vi "Magnetic Sweep 1.9c.vi"() -> ()   [LabVIEW 2011]
panel:
  in  "Save":bool
  out "file position4":errorcluster
  out "file position3":errorcluster
  out "file position2":errorcluster
  out "File position1":errorcluster
  out "Initial Temperature check":errorcluster
  out "Status":i32
  out "Loop end check":errorcluster
  out "Parameter setup":errorcluster
  out "Resistance check":errorcluster
  out "Start ramping":errorcluster
  out "Cell temperature\ncheck":errorcluster
  out "Initial Temp\nCheck":errorcluster
  out "Current time":timestamp format="%<%I:%M:%S %p\n%x>T"
  out "x .and. y?":bool
  in  "Initial\nTemperature":dbl
  out "Heater":bool
  out "Persistent switch ready":bool
  out "Initial check":errorcluster
  in  "Temperature\nlower limite":dbl
  out "Ramping rate command":string
  out "Target field command":string
  out "String":string="Persistent switch is not on"
  in  "Set parameter":bool
  out "status":string
  out "PID command":string
  out "setpoint command":string
  out "setpoint":dbl
  in  "stop":bool
  in  "Contour plot (ramp down)":path
  in  "Raw data (ramp down)":path
  out "Elapsed Time (s)":dbl
  out "Iteration":i32
  out "Zero field reached":bool
  out "Target field reached":bool
  in  "Temperature\nupper limite":dbl
  in  "Temperature\nramping step":dbl
  in  "Heater range":i16(ring) items=["High", "Medium", "Low"]
  in  "D gain":dbl
  in  "I gain":dbl
  in  "P gain":dbl
  in  "Contour plot (ramp up)":path
  in  "Timer":bool caption="Reset"
  in  "Raw data (ramp  up)":path
  out "Current Resistance":string
  out "Current Temperature":string
  out "Current Field":string
  in  "Sweep":bool
  in  "Magnetic field\nRamp rate":dbl
  in  "Traget Field":dbl
  out "Init Response":string
  in  "Update":bool
  in  "P Switch on/off":bool
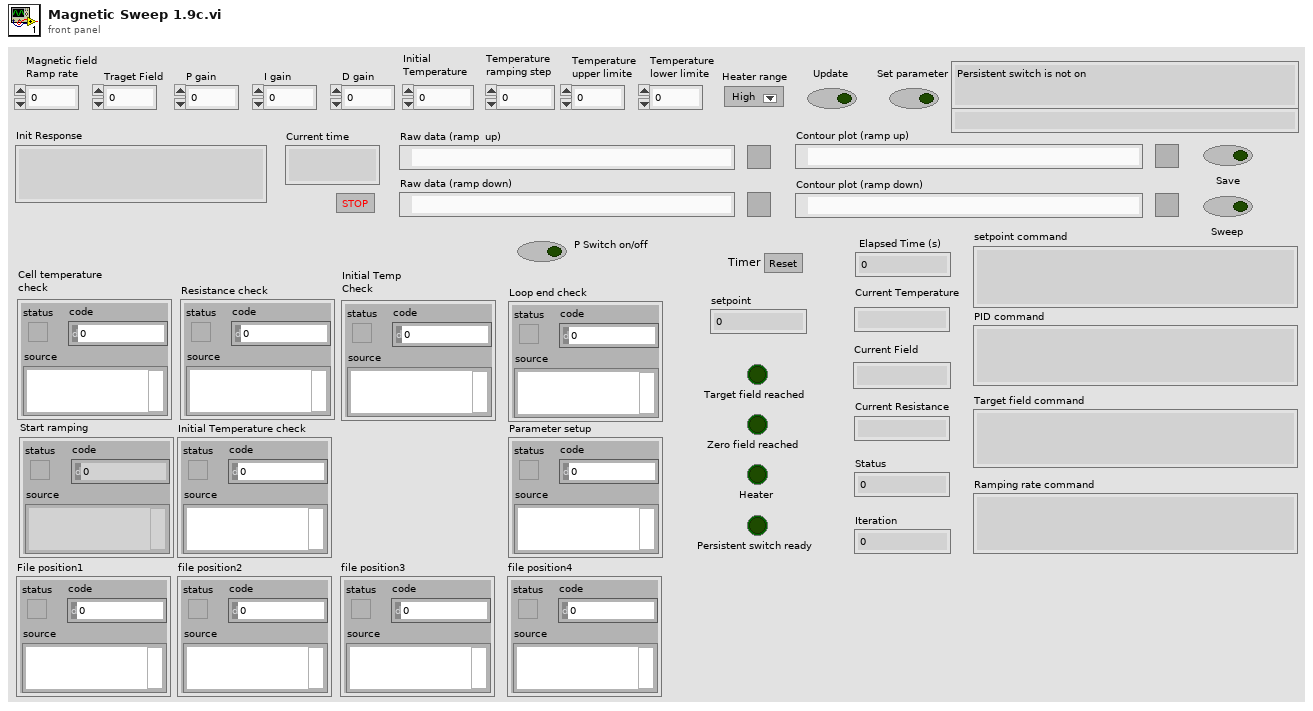
[diagram p1: front panel]
types:
  T1 = enum16{"open", "replace", "create", "open or create", "replace or create", "replace or create with confirmation"}
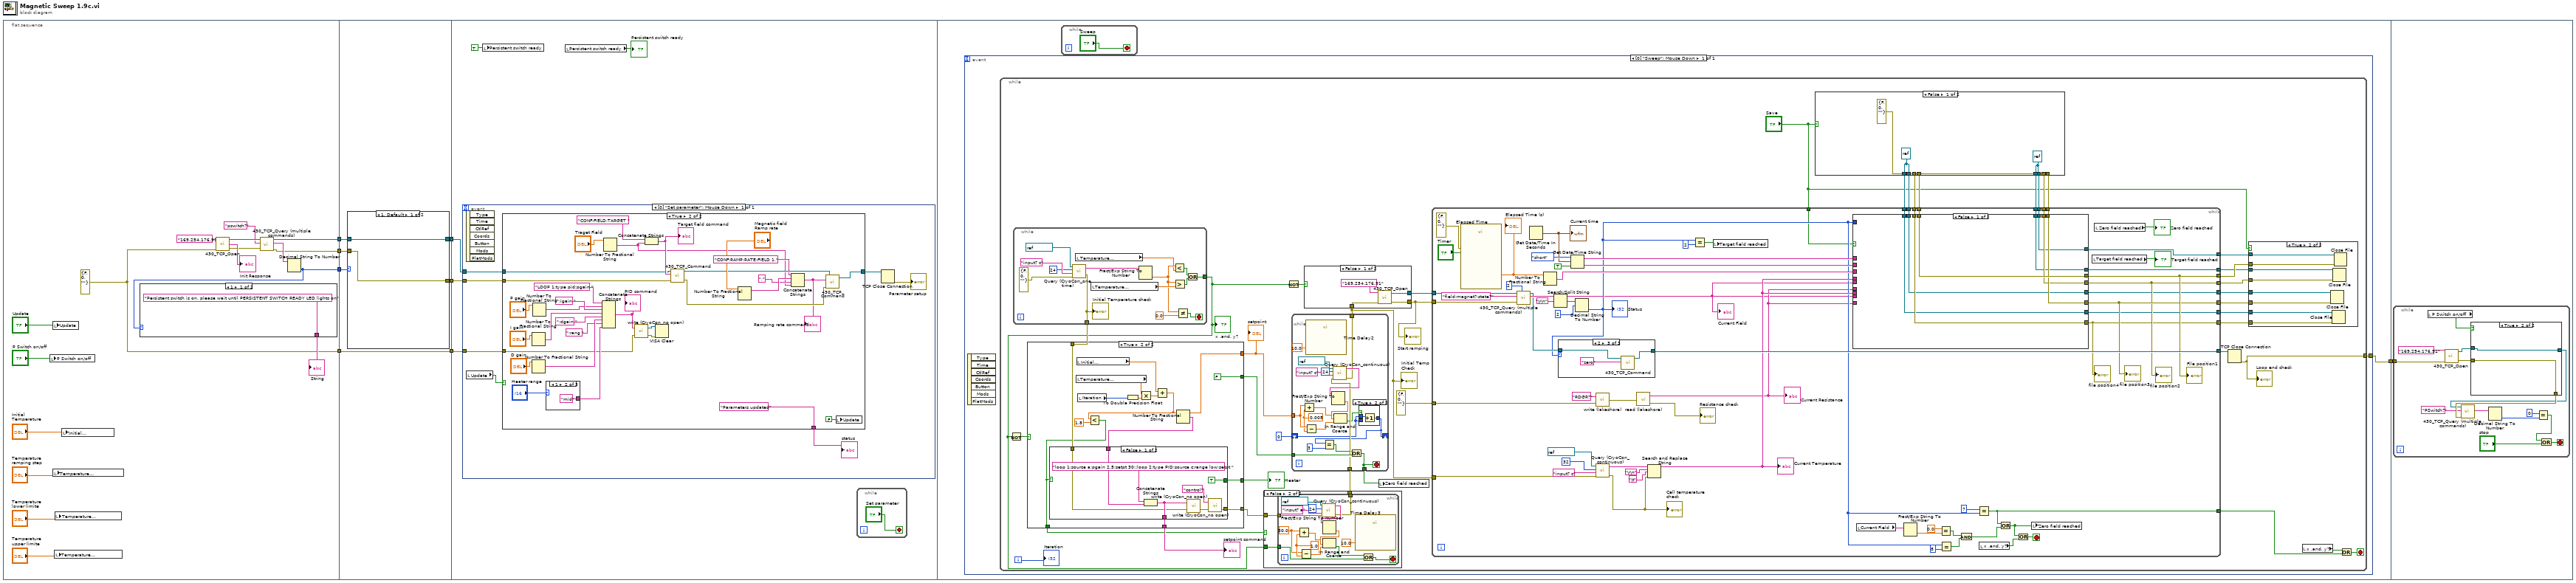
[diagram p0: block diagram]
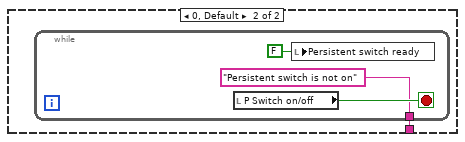
[diagram p2: hidden frame]
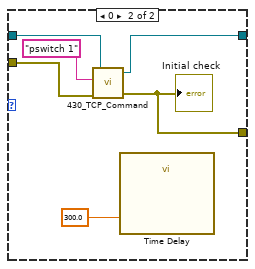
[diagram p3: hidden frame]
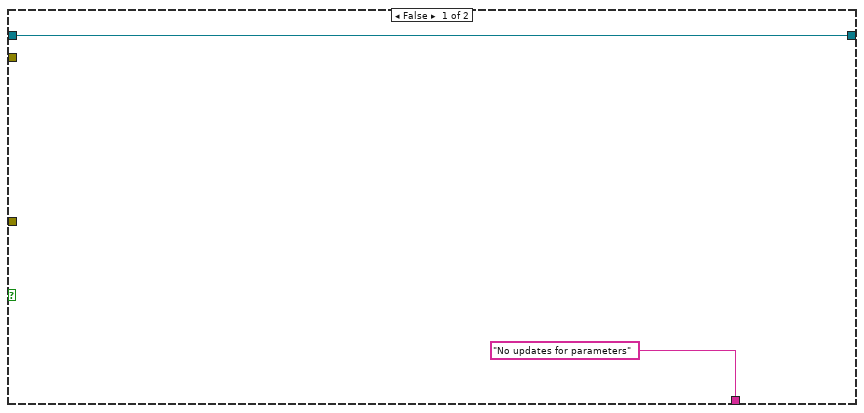
[diagram p4: hidden frame]
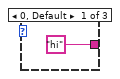
[diagram p5: hidden frame]
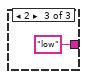
[diagram p6: hidden frame]
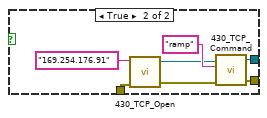
[diagram p7: hidden frame]
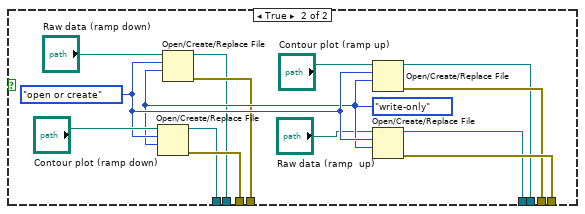
[diagram p9: hidden frame]
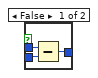
[diagram p11: hidden frame]
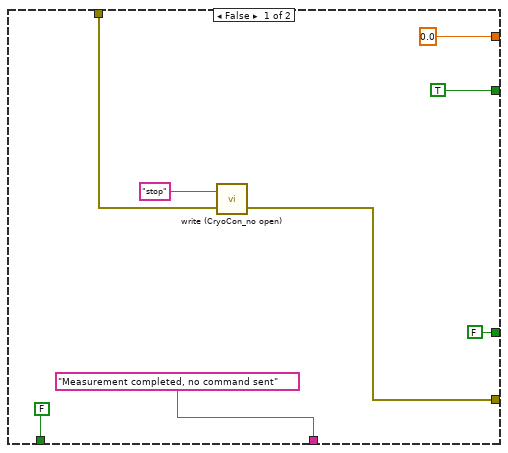
[diagram p12: hidden frame]
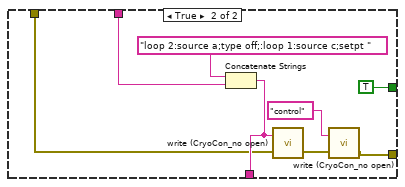
[diagram p13: hidden frame]
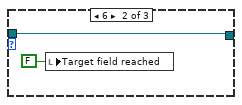
[diagram p15: hidden frame]
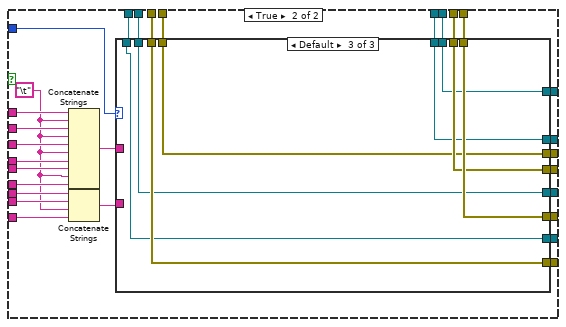
[diagram p16: hidden frame]
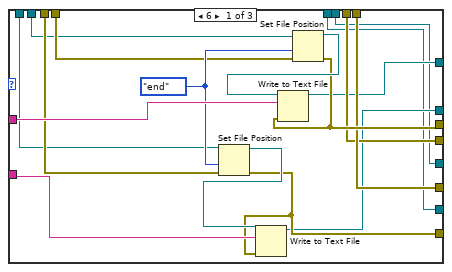
[diagram p17: hidden frame]
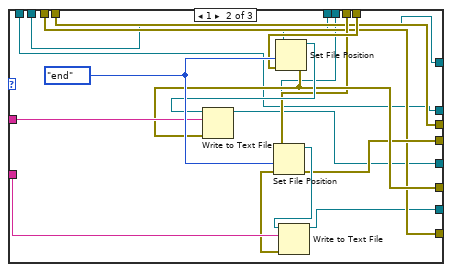
[diagram p18: hidden frame]
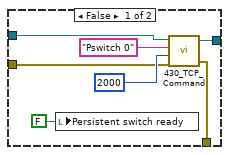
[diagram p19: hidden frame]
diagram:
  n1 = flat-sequence {
    tunnel: [w14] -> w8
    tunnel: [w13] -> w6
    tunnel: [w11] -> w5
    tunnel: [w9] -> w2
    tunnel: w8 -> [w36]
    tunnel: [w35] -> w7
    tunnel: w6 -> [w34]
    tunnel: w5 -> [w33]
    tunnel: [w32] -> w4
    tunnel: [w31] -> w3
    tunnel: w2 -> [w31]
    tunnel: w7 -> [w47]
    tunnel: w4 -> [w46]
    tunnel: w3 -> [w45]
    tunnel: [w95] -> w1
    tunnel: w1 -> [w422]
    frame #0 {
      w9 = errorcluster {"status"=FALSE, "code"=0, "source"=""} ("error in (no error)")
      n2 = local write "P Switch on/off"("P Switch on/off") -> ()
      n3 = local write "Update"("Update") -> ()
      n4 = local write "Temperature\nramping step"("Temperature\nramping step") -> ()
      n5 = local write "Temperature\nupper limite"("Temperature\nupper limite") -> ()
      n6 = local write "Temperature\nlower limite"("Temperature\nlower limite") -> ()
      n7 = local write "Initial\nTemperature"("Initial\nTemperature") -> ()
      n8 = call "430_TCP_Open.vi"("IP Address"="169.254.176.91", "error in (no error)"=w9) -> ("connection ID"=w20:refnum<k5>, "Init Response"=→"Init Response":string, "error out"=w19:errorcluster)  [unwired: 4 in]
      n9 = call "430_TCP_Query (multiple commands).vi"("error in (no error)"=w19, "Command"="pswitch?", "connection ID"=w20) -> ("error out"=w11:errorcluster, "Response"=w17:string, "connection ID out"=w14:refnum<k5>)  [unwired: 4 in, 2 out]
      n10 = Decimal String To Number(string=w17) -> (number=w13:i32)  [unwired: 2 in, 1 out]
      n11 = case shown="1" w13 {
        tunnel: ["Persistent switch is on, please wait until PERSISTENT SWITCH READY LED lights on" w27] -> w16
        frame 1 {
        }
        frame 0, Default {
          n12 = while {
            tunnel: ["Persistent switch is not on"] -> w27
            stop <- w30 stop-if-true
            n13 = local read "P Switch on/off"() -> (w30:bool)
            n14 = local write "Persistent switch ready"(FALSE ("Persistent switch ready")) -> ()
          }
        }
      }
      "String" <- w16
    }
    frame #1 {
      n15 = case shown="1, Default" w34 {
        tunnel: w36 -> [w38 w44]
        tunnel: [w38 w43] -> w35
        tunnel: w33 -> [w37 w40]
        tunnel: [w37 w39] -> w32
        frame 1, Default {
        }
        frame 0 {
          n16 = call "430_TCP_Command.vi"("error in (no error)"=w40, "Command"="pswitch 1", "connection ID"=w44) -> ("error out"=w39:errorcluster, "connection ID out"=w43:refnum<k5>)  [unwired: 1 in, 1 out]
          "Initial check" <- w39
          n17 = call "Time Delay"("Delay Time (s)"=300.0) -> ()  [unwired: 10 in, 1 out]
        }
      }
    }
    frame #2 {
      n18 = event shown="[0] \"Set parameter\": Mouse Down" {
        selector: _ -> [_]
        dyn-events: _ -> [_]
        timeout: _ -> [_]
        tunnel: w47 -> [w57]
        tunnel: w46 -> [w52]
        tunnel: w45 -> [w51]
        event "Set parameter": Mouse Down {
          n19 = event-data() -> ()  [unwired: 1 in, 7 out]
          n20 = local read "Update"() -> (w55:bool)
          n21 = case shown="True" w55 {
            tunnel: w57 -> [w58 w89]
            tunnel: ["No updates for parameters" ("String") "Parameters updated" ("String")] -> w56
            tunnel: [w58 w64] -> w54
            tunnel: w52 -> [_ w61]
            tunnel: w51 -> [_ w60]
            frame False {
            }
            frame True {
              n22 = Number To Fractional String(number="I gain") -> (F-format string=w72:string)  [unwired: 3 in]
              n23 = Number To Fractional String(number="D gain") -> (F-format string=w70:string)  [unwired: 3 in]
              n24 = Number To Fractional String(number="P gain") -> (F-format string=w73:string)  [unwired: 3 in]
              n25 = case shown="1" "Heater range" {
                tunnel: ["hi" "mid" "low"] -> w66
                frame 0, Default {
                }
                frame 1 {
                }
                frame 2 {
                }
              }
              n26 = Concatenate Strings("LOOP 1:type pid;pgain " ("write buffer"), w73, ";igain " ("string"), w72, ";dgain " ("string"), w70, ";rang " ("string"), w66) -> (w69:string)
              "PID command" <- w69
              n27 = Number To Fractional String(number="Traget Field") -> (F-format string=w79:string)  [unwired: 3 in]
              n28 = call "write (CryoCon_no open).vi"("error in (no error)"=w60, "write buffer"=w69) -> ("error out"=w63:errorcluster, "VISA resource name out"=w62:refnum<visa-resource-name>)
              n29 = Concatenate Strings("CONF:FIELD:TARGET ", w79) -> (w90:string)
              "Target field command" <- w90
              n30 = VISA Clear(VISA resource name=w62, error in (no error)=w63) -> ()  [unwired: 2 out]
              n31 = call "430_TCP_Command.vi"("error in (no error)"=w61, "Command"=w90, "connection ID"=w89) -> ("error out"=w88:errorcluster, "connection ID out"=w84:refnum<k5>)  [unwired: 1 in, 1 out]
              n32 = Number To Fractional String(number="Magnetic field\nRamp rate") -> (F-format string=w82:string)  [unwired: 3 in]
              n33 = Concatenate Strings("CONF:RAMP:RATE:FIELD 1," ("string"), w82, "," ("string"), w79) -> (w85:string)
              "Ramping rate command" <- w85
              n34 = call "430_TCP_Command.vi"("error in (no error)"=w88, "Command"=w85, "connection ID"=w84) -> ("connection ID out"=w64:refnum<k5>)  [unwired: 1 in, 2 out]
              n35 = local write "Update"(FALSE ("Update")) -> ()
            }
          }
          "status" <- w56
          n36 = TCP Close Connection(connection ID=w54) -> (error out=→"Parameter setup":errorcluster)  [unwired: 2 in, 1 out]
        }
      }
      n37 = local write "Persistent switch ready"(TRUE ("Persistent switch ready")) -> ()
      n38 = local read "Persistent switch ready"() -> (→"Persistent switch ready":bool)
      n39 = while {
        stop <- "Set parameter" stop-if-true
      }
    }
    frame #3 {
      n40 = event shown="[0] \"Sweep\": Mouse Down" {
        selector: _ -> [_]
        dyn-events: _ -> [_]
        timeout: _ -> [_]
        tunnel: [w97] -> w95
        event "Sweep": Mouse Down {
          n41 = event-data() -> ()  [unwired: 1 in, 7 out]
          n42 = while {
            tunnel: [w120] -> w97
            i -> [w136]
            stop <- w132 stop-if-true
            n43 = while {
              tunnel: [w148] -> w130
              tunnel: [w138] -> w98
              stop <- w144 stop-if-true
              n44 = call "Query (CryoCon_one time).vi"("error in (no error)"=errorcluster {"status"=FALSE, "code"=0, "source"=""}, "write buffer"="input? c", "byte count"=u32 24, "VISA resource name 2"=refnum<visa-resource-name> "COM3") -> ("error out"=w148:errorcluster, "read buffer"=w149:string)
              "Initial Temperature check" <- w148
              n45 = local read "Temperature\nlower limite"() -> (w141:dbl)
              n46 = local read "Temperature\nupper limite"() -> (w151:dbl)
              n47 = Fract/Exp String To Number(string=w149) -> (number=w142:dbl)  [unwired: 3 in, 1 out]
              n48 = Less?(x=w142, y=w141) -> (x < y?=w139:bool)
              n49 = Greater?(x=w142, y=w151) -> (0:w140:bool)
              n50 = Not Equal?(x=w142, y=0.0) -> (x != y?=w144:bool)
              n51 = Or(x=w139, y=w140) -> (x .or. y?=w138:bool)
            }
            "x .and. y?" <- w98
            n52 = Not(x=w98) -> (.not. x?=w129:bool)
            n53 = case shown="True" w129 {
              tunnel: [w232 w247] -> w124
              tunnel: [0.0 w245] -> w137
              tunnel: ["Measurement completed, no command sent" w248] -> w128
              tunnel: [TRUE FALSE] -> w135
              tunnel: w130 -> [w234 w241]
              tunnel: [FALSE ("Heater") w240] -> w126
              tunnel: [FALSE w239] -> w125
              frame False {
                n54 = call "write (CryoCon_no open).vi"("error in (no error)"=w234, "write buffer"="stop") -> ("error out"=w232:errorcluster)  [unwired: 1 out]
              }
              frame True {
                n55 = local read "Temperature\nramping step"() -> (w250:dbl)
                n56 = local read "Initial\nTemperature"() -> (w243:dbl)
                n57 = local read "Iteration"() -> (w242:i32)
                n58 = To Double Precision Float(number=w242) -> (double precision float=w249:dbl)
                n59 = Multiply(x=w250, y=w249) -> (x*y=w251:dbl)
                n60 = Add(x=w243, y=w251) -> (x+y=w245:dbl)
                n61 = Less?(x=w245, y=1.8) -> (x < y?=w239:bool)
                n62 = Number To Fractional String(number=w245) -> (F-format string=w252:string)  [unwired: 3 in]
                n63 = case shown="False" w239 {
                  tunnel: w252 -> [w259 w267]
                  tunnel: [w256 w266] -> w248
                  tunnel: [w258 w265] -> w247
                  tunnel: w241 -> [w253 w262]
                  tunnel: [TRUE ("Heater") TRUE ("Heater")] -> w240
                  frame False {
                    n64 = Concatenate Strings("loop 1:source a;pgain 2.5;setpt 30;:loop 2:type PID;source c;range low;setpt " ("write buffer"), w259) -> (w256:string)
                    n65 = call "write (CryoCon_no open).vi"("error in (no error)"=w253, "write buffer"=w256) -> ("error out"=w255:errorcluster)  [unwired: 1 out]
                    n66 = call "write (CryoCon_no open).vi"("error in (no error)"=w255, "write buffer"="control") -> ("error out"=w258:errorcluster)  [unwired: 1 out]
                  }
                  frame True {
                    n67 = Concatenate Strings("loop 2:source a;type off;:loop 1:source c;setpt " ("write buffer"), w267) -> (w266:string)
                    n68 = call "write (CryoCon_no open).vi"("error in (no error)"=w262, "write buffer"=w266) -> ("error out"=w264:errorcluster)  [unwired: 1 out]
                    n69 = call "write (CryoCon_no open).vi"("error in (no error)"=w264, "write buffer"="control") -> ("error out"=w265:errorcluster)  [unwired: 1 out]
                  }
                }
              }
            }
            "setpoint" <- w137
            "setpoint command" <- w128
            "Heater" <- w126
            n70 = case shown="False" w125 {
              tunnel: w124 -> [w188 w191]
              tunnel: [w188 w190] -> w123
              tunnel: w98 -> [_ w189]
              frame True {
              }
              frame False {
                n71 = while {
                  tunnel: w191 -> [w203]
                  tunnel: [w194] -> w190
                  tunnel: w189 -> [w192]
                  stop <- w195 stop-if-true
                  w197 = 30.0 ("x")
                  w198 = 1.0 ("y")
                  n72 = Add(x=w197, y=w198) -> (x+y=w200:dbl)
                  n73 = Subtract(x=w197, y=w198) -> (x-y=w199:dbl)
                  n74 = call "Query (CryoCon_continuous).vi"("error in (no error)"=w203, "write buffer"="input? a", "byte count"=u32 24, "VISA resource name"=refnum<visa-resource-name> "COM3" ("VISA resource name 2")) -> ("error out"=w194:errorcluster, "read buffer"=w202:string)  [unwired: 1 out]
                  n75 = Fract/Exp String To Number(string=w202) -> (number=w201:dbl)  [unwired: 3 in, 1 out]
                  n76 = In Range and Coerce(upper limit=w200, x=w201, lower limit=w199) -> (In Range?=w196:bool)  [unwired: 1 out]
                  n77 = call "Time Delay3"("Delay Time (s)"=10.0) -> ()  [unwired: 10 in, 1 out]
                  n78 = Or(x=w196, y=w192) -> (x .or. y?=w195:bool)
                }
              }
            }
            n79 = Not(x=w98) -> (.not. x?=w99:bool)
            n80 = while {
              tunnel: w137 -> [w224]
              tunnel: w135 -> [w216]
              tunnel: [w215] -> w100
              tunnel: [w214] -> w127
              tunnel: w123 -> [w213]
              shift-right: [w211] -> _
              shift-left: 0 -> [w208]
              stop <- w214 stop-if-true
              w221 = 0.005 ("y")
              n81 = Add(x=w224, y=w221) -> (x+y=w223:dbl)
              n82 = Subtract(x=w224, y=w221) -> (x-y=w222:dbl)
              n83 = call "Time Delay2"("Delay Time (s)"=10.0) -> ()  [unwired: 10 in, 1 out]
              n84 = call "Query (CryoCon_continuous).vi"("error in (no error)"=w213, "write buffer"="input? c", "byte count"=u32 24, "VISA resource name"=refnum<visa-resource-name> "COM3" ("VISA resource name 2")) -> ("error out"=w215:errorcluster, "read buffer"=w218:string)  [unwired: 1 out]
              n85 = Fract/Exp String To Number(string=w218) -> (number=w225:dbl)  [unwired: 3 in, 1 out]
              n86 = In Range and Coerce(upper limit=w223, x=w225, lower limit=w222) -> (In Range?=w212:bool)  [unwired: 1 out]
              n87 = case shown="True" w212 {
                tunnel: w208 -> [w228 w229]
                tunnel: [w226 w230] -> w211
                tunnel: w208 -> [w227 _]
                frame False {
                  n88 = Subtract(x=w228, y=w227) -> (x-y=w226:i32)
                }
                frame True {
                  n89 = Increment(x=w229) -> (x+1=w230:i32)
                }
              }
              n90 = Equal?(x=w211, y=3) -> (x = y?=w210:bool)
              n91 = Or(x=w210, y=w216) -> (x .or. y?=w214:bool)
            }
            "Initial Temp\nCheck" <- w100
            n92 = case shown="False" w99 {
              tunnel: [w154 w161] -> w134
              tunnel: [w152 w158] -> w122
              tunnel: w100 -> [w153 w156]
              frame False {
                n93 = call "430_TCP_Open.vi"("IP Address"="169.254.176.91", "error in (no error)"=w153) -> ("connection ID"=w154:refnum<k5>, "error out"=w152:errorcluster)  [unwired: 4 in, 1 out]
              }
              frame True {
                n94 = call "430_TCP_Open.vi"("IP Address"="169.254.176.91", "error in (no error)"=w156) -> ("connection ID"=w159:refnum<k5>, "error out"=w160:errorcluster)  [unwired: 4 in, 1 out]
                n95 = call "430_TCP_Command.vi"("error in (no error)"=w160, "Command"="ramp", "connection ID"=w159) -> ("error out"=w158:errorcluster, "connection ID out"=w161:refnum<k5>)  [unwired: 1 in, 1 out]
              }
            }
            "Start ramping" <- w122
            n96 = local write "Zero field reached"(w127) -> ()
            n97 = case shown="False" "Save" {
              tunnel: [w173 w181] -> w115
              tunnel: [w173 w180] -> w114
              tunnel: [w173 w179] -> w117
              tunnel: [w173 w178] -> w116
              tunnel: [w172 w177] -> w109
              tunnel: [w172 w176] -> w108
              tunnel: [w171 w175] -> w107
              tunnel: [w171 w174] -> w106
              frame False {
                w171 = refnum<file> refnum ("refnum out")
                w172 = refnum<file> refnum ("refnum out")
                w173 = errorcluster {"status"=FALSE, "code"=0, "source"=""} ("error out")
              }
              frame True {
                w184 = enum16{"read/write", "read-only", "write-only"}."write-only" ("access (0:read/write)")
                w185 = T1."open or create" ("operation (0:open)")
                n98 = Open/Create/Replace File(file path (use dialog)="Contour plot (ramp down)", operation (0:open)=w185, access (0:read/write)=w184) -> (refnum out=w176:refnum<file>, error out=w180:errorcluster)  [unwired: 3 in, 1 out]
                n99 = Open/Create/Replace File(file path (use dialog)="Raw data (ramp down)", operation (0:open)=w185, access (0:read/write)=w184) -> (refnum out=w177:refnum<file>, error out=w181:errorcluster)  [unwired: 3 in, 1 out]
                n100 = Open/Create/Replace File(file path (use dialog)="Contour plot (ramp up)", operation (0:open)=w185, access (0:read/write)=w184) -> (refnum out=w174:refnum<file>, error out=w178:errorcluster)  [unwired: 3 in, 1 out]
                n101 = Open/Create/Replace File(file path (use dialog)="Raw data (ramp  up)", operation (0:open)=w185, access (0:read/write)=w184) -> (refnum out=w175:refnum<file>, error out=w179:errorcluster)  [unwired: 3 in, 1 out]
              }
            }
            n102 = while {
              tunnel: w134 -> [w331]
              tunnel: [w318] -> w133
              tunnel: w122 -> [w312]
              tunnel: [w311] -> w121
              tunnel: errorcluster {"status"=FALSE, "code"=0, "source"=""} ("error in (no error)") -> [w291]
              tunnel: w117 -> [w289]
              tunnel: w116 -> [w288]
              tunnel: w115 -> [w287]
              tunnel: w114 -> [w286]
              tunnel: [w285] -> w113
              tunnel: [w277] -> w112
              tunnel: [w284] -> w111
              tunnel: [w278] -> w110
              tunnel: w109 -> [w283]
              tunnel: w108 -> [w282]
              tunnel: w107 -> [w281]
              tunnel: w106 -> [w280]
              tunnel: "Save" -> [w279]
              tunnel: [w276] -> w104
              tunnel: [w275] -> w103
              tunnel: [w274] -> w102
              tunnel: [w273] -> w101
              tunnel: w100 -> [w272]
              stop <- w320 stop-if-true
              n103 = call "Elapsed Time"("Reset"="Timer", "error in (no error)"=errorcluster {"status"=FALSE, "code"=0, "source"=""}) -> ("Elapsed Time (s)"=w329:dbl)  [unwired: 10 in, 7 out]
              "Elapsed Time (s)" <- w329
              n104 = call "430_TCP_Query (multiple commands).vi"("Number of\nquerys"=2 ("Number of\nquerys"), "error in (no error)"=w312, "Command"="field:magnet?;state?", "connection ID"=w331) -> ("Response"=w301:string, "connection ID out"=w299:refnum<k5>)  [unwired: 3 in, 3 out]
              n105 = Get Date/Time In Seconds() -> (seconds since 1Jan1904=w309:timestamp)
              "Current time" <- w309
              n106 = Number To Fractional String(number=w329) -> (F-format string=w304:string)  [unwired: 3 in]
              n107 = Search/Split String(string=w301, search string/char (-)="\r\n") -> (substring before match=w269:string, match + rest of string=w295:string)  [unwired: 1 in, 1 out]
              "Current Field" <- w269
              n108 = Get Date/Time String(date format (0)=enum16{"short", "long", "abbreviated"}."short", seconds (now)=w309, want seconds? (F)=TRUE) -> (date string=w306:string, time string=w305:string)
              n109 = Decimal String To Number(string=w295, offset=2) -> (number=w294:i32)  [unwired: 1 in, 1 out]
              "Status" <- w294
              n110 = case shown="2" w294 {
                tunnel: [w337 w338 w341] -> w311
                tunnel: w299 -> [w337 w338 w340]
                frame 0, Default {
                }
                frame 6 {
                  n111 = local write "Target field reached"(FALSE ("Target field reached")) -> ()
                }
                frame 2 {
                  n112 = call "430_TCP_Command.vi"("Command"="zero", "connection ID"=w340) -> ("connection ID out"=w341:refnum<k5>)  [unwired: 2 in, 2 out]
                }
              }
              n113 = call "write (lakeshore).vi"("error in (no error)"=w291, "write buffer"="RDGR?") -> ("error out"=w335:errorcluster)
              n114 = call "Query (CryoCon_continuous).vi"("error in (no error)"=w272, "write buffer"="input? c", "byte count"=u32 32, "VISA resource name"=refnum<visa-resource-name> "COM3") -> ("error out"=w270:errorcluster, "read buffer"=w298:string)  [unwired: 1 out]
              "Cell temperature\ncheck" <- w270
              n115 = call "read (lakeshore).vi"("error in (no error)"=w335) -> ("read buffer"=w292:string, "error out"=→"Resistance check":errorcluster)
              "Current Resistance" <- w292
              n116 = Search and Replace String(input string=w298, search string="\r\n", replace string="\t", error in=w270) -> (result string=w303:string)  [unwired: 4 in, 3 out]
              "Current Temperature" <- w303
              n117 = Equal?(x=w294, y=2) -> (x = y?=w330:bool)
              n118 = local write "Target field reached"(w330) -> ()
              n119 = case shown="False" w279 {
                tunnel: w294 -> [_ w379]
                tunnel: w306 -> [_ w376]
                tunnel: w305 -> [_ w375]
                tunnel: w304 -> [_ w374]
                tunnel: w303 -> [_ w373]
                tunnel: w269 -> [_ w372]
                tunnel: w292 -> [_ w365]
                tunnel: w303 -> [_ w371]
                tunnel: w269 -> [_ w370]
                tunnel: [w347 w369] -> w278
                tunnel: [w348 w368] -> w284
                tunnel: [w349 w367] -> w277
                tunnel: w292 -> [_ w366]
                tunnel: w289 -> [w348 w363]
                tunnel: w288 -> [w347 w362]
                tunnel: w287 -> [w350 w361]
                tunnel: w286 -> [w349 w360]
                tunnel: [w350 w359] -> w285
                tunnel: w283 -> [w344 w358]
                tunnel: w282 -> [w343 w357]
                tunnel: w281 -> [w345 w356]
                tunnel: w280 -> [w346 w355]
                tunnel: [w346 w354] -> w276
                tunnel: [w345 w353] -> w275
                tunnel: [w344 w352] -> w274
                tunnel: [w343 w351] -> w273
                frame False {
                }
                frame True {
                  w364 = "\t"
                  n120 = Concatenate Strings(w376, w364, w375, w364, w374, w364, w373, w372, w364, w365) -> (w378:string)
                  n121 = Concatenate Strings(w371, w370, w364, w366) -> (w377:string)
                  n122 = case shown="Default" w379 {
                    tunnel: w378 -> [w396 w412 _]
                    tunnel: w377 -> [w395 w411 _]
                    tunnel: [w386 w407 w420] -> w369
                    tunnel: [w387 w408 w421] -> w368
                    tunnel: [w391 w404 w418] -> w367
                    tunnel: w363 -> [w387 w406 w421]
                    tunnel: w362 -> [w386 w405 w420]
                    tunnel: w361 -> [w390 w403 w419]
                    tunnel: w360 -> [w389 w404 w418]
                    tunnel: [w388 w403 w419] -> w359
                    tunnel: w358 -> [w385 w398 w415]
                    tunnel: w357 -> [w384 w397 w414]
                    tunnel: w356 -> [w380 w402 w416]
                    tunnel: w355 -> [w381 w401 w417]
                    tunnel: [w383 w398 w417] -> w354
                    tunnel: [w382 w397 w416] -> w353
                    tunnel: [w381 w400 w415] -> w352
                    tunnel: [w380 w399 w414] -> w351
                    frame 6 {
                      w394 = enum16{"start", "end", "current"}."end" ("from (0:start)")
                      n123 = Set File Position(refnum=w384, from (0:start)=w394, error in=w389) -> (refnum out=w392:refnum<file>, error out=w391:errorcluster)  [unwired: 1 in]
                      n124 = Write to Text File(file (use dialog)=w392, text=w395, error in=w391) -> (refnum out=w382:refnum<file>)  [unwired: 1 in, 2 out]
                      n125 = Set File Position(refnum=w385, from (0:start)=w394, error in=w390) -> (refnum out=w393:refnum<file>, error out=w388:errorcluster)  [unwired: 1 in]
                      n126 = Write to Text File(file (use dialog)=w393, text=w396, error in=w388) -> (refnum out=w383:refnum<file>)  [unwired: 1 in, 2 out]
                    }
                    frame 1 {
                      w413 = enum16{"start", "end", "current"}."end" ("from (0:start)")
                      n127 = Set File Position(refnum=w401, from (0:start)=w413, error in=w405) -> (refnum out=w409:refnum<file>, error out=w407:errorcluster)  [unwired: 1 in]
                      n128 = Set File Position(refnum=w402, from (0:start)=w413, error in=w406) -> (refnum out=w410:refnum<file>, error out=w408:errorcluster)  [unwired: 1 in]
                      n129 = Write to Text File(file (use dialog)=w410, text=w412, error in=w408) -> (refnum out=w400:refnum<file>)  [unwired: 1 in, 2 out]
                      n130 = Write to Text File(file (use dialog)=w409, text=w411, error in=w407) -> (refnum out=w399:refnum<file>)  [unwired: 1 in, 2 out]
                    }
                    frame Default {
                    }
                  }
                }
              }
              "file position4" <- w277
              "file position3" <- w284
              "file position2" <- w278
              "File position1" <- w285
              n131 = local read "Current Field"() -> (w314:string)
              n132 = Fract/Exp String To Number(string=w314) -> (number=w315:dbl)  [unwired: 3 in, 1 out]
              n133 = Equal?(x=0.0, y=w315) -> (x = y?=w323:bool)
              n134 = Equal?(x=w294, y=8) -> (x = y?=w324:bool)
              n135 = And(x=w323, y=w324) -> (x .and. y?=w322:bool)
              n136 = Equal?(x=7, y=w294) -> (x = y?=w318:bool)
              n137 = local read "x .and. y?"() -> (w319:bool)
              n138 = Or(x=w318, y=w322) -> (x .or. y?=w321:bool)
              n139 = Or(x=w321, y=w319) -> (x .or. y?=w320:bool)
              n140 = local write "Zero field reached"(w321) -> ()
              n141 = local read "Target field reached"() -> (→"Target field reached":bool)
              n142 = local read "Zero field reached"() -> (→"Zero field reached":bool)
            }
            n143 = TCP Close Connection(connection ID=w121) -> (error out=w120:errorcluster)  [unwired: 2 in, 1 out]
            "Loop end check" <- w120
            n144 = case shown="True" "Save" {
              tunnel: w113 -> [_ w170]
              tunnel: w112 -> [_ w169]
              tunnel: w111 -> [_ w168]
              tunnel: w110 -> [_ w167]
              tunnel: w104 -> [_ w166]
              tunnel: w103 -> [_ w165]
              tunnel: w102 -> [_ w164]
              tunnel: w101 -> [_ w163]
              frame False {
              }
              frame True {
                n145 = Close File(refnum=w164, error in=w168) -> ()  [unwired: 2 out]
                n146 = Close File(refnum=w163, error in=w169) -> ()  [unwired: 2 out]
                n147 = Close File(refnum=w165, error in=w167) -> ()  [unwired: 2 out]
                n148 = Close File(refnum=w166, error in=w170) -> ()  [unwired: 2 out]
              }
            }
            n149 = local read "x .and. y?"() -> (w131:bool)
            n150 = Or(x=w131, y=w133) -> (x .or. y?=w132:bool)
            "Iteration" <- w136
          }
        }
      }
      n151 = while {
        stop <- "Sweep" stop-if-true
      }
    }
    frame #4 {
      n152 = while {
        tunnel: w422 -> [w423]
        stop <- w427 stop-if-true
        n153 = local read "P Switch on/off"() -> (w436:bool)
        n154 = call "430_TCP_Open.vi"("IP Address"="169.254.176.91", "error in (no error)"=w423) -> ("connection ID"=w426:refnum<k5>, "error out"=w425:errorcluster)  [unwired: 4 in, 1 out]
        n155 = case shown="True" w436 {
          tunnel: [w440 w444] -> w434
          tunnel: [w439 w445] -> w433
          tunnel: w426 -> [w438 w445]
          tunnel: w425 -> [w437 w444]
          frame False {
            n156 = local write "Persistent switch ready"(FALSE ("Persistent switch ready")) -> ()
            n157 = call "430_TCP_Command.vi"("error in (no error)"=w437, "Timeout"=2000, "Command"="Pswitch 0", "connection ID"=w438) -> ("error out"=w440:errorcluster, "connection ID out"=w439:refnum<k5>)  [unwired: 1 out]
          }
          frame True {
          }
        }
        n158 = call "430_TCP_Query (multiple commands).vi"("error in (no error)"=w434, "Command"="PSwitch?", "connection ID"=w433) -> ("Response"=w431:string)  [unwired: 4 in, 4 out]
        n159 = Decimal String To Number(string=w431) -> (number=w430:i32)  [unwired: 2 in, 1 out]
        n160 = Equal?(x=0, y=w430) -> (x = y?=w428:bool)
        n161 = Or(x=w428, y="stop") -> (x .or. y?=w427:bool)
      }
    }
  }
